vi "VI Server_GetComboBoxValuesArray.vi"(7 "Label":string, 8 "error in":errorcluster, 11 "VI Server Cluster":T1) -> (0 "error out":errorcluster, 1 "Control Reference":refnum<vi>, 3 "VI Server Custer.DUP":T1={"Labels"=["Label", "Size", "Font", "Heght", "Width", "Ledding Denominator", "Ledding Nominator", "Label Number", "Microstep Resolution", "X", "Y", "Z", "Italic?", "Underlined?"], "Refs"=[], "VI Ref"=refnum}, 4 "Strings[]":string[](array[string]), 6 "Values[]":string[](array[string]))   [LabVIEW 2020, in "VI Server Toolkit LV2013.lvlib"]
doc: "Returns array of item names and array of the corresponding values."
uses:
  VI Server Toolkit LV2013.lvlib
  VI Server_TypeDefs/VI Server_RefsCluster.ctl
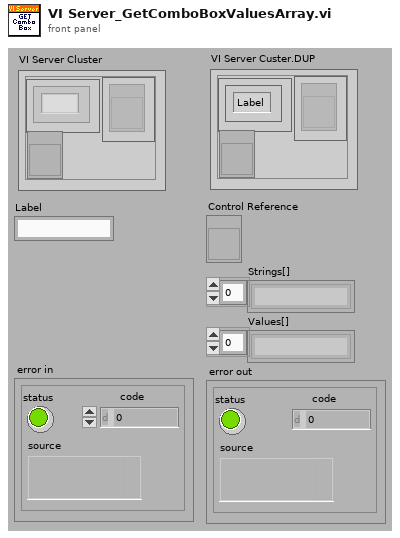
[diagram p1: front panel]
types:
  T1 = typedef "VI Server_RefsCluster.ctl" = cluster{"Labels":string[], "Refs":refnum<vi>[], "VI Ref":refnum<vi>}
  T2 = typedef "LVComboBoxStrsAndValuesArrayTypeDef.ctl" = cluster{"String":string, "Value":string}[]
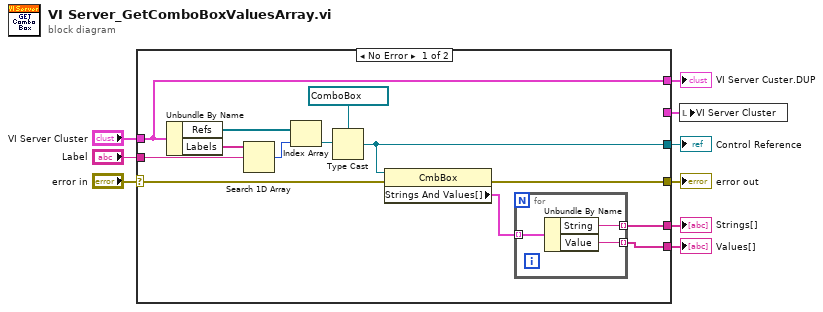
[diagram p0: block diagram]
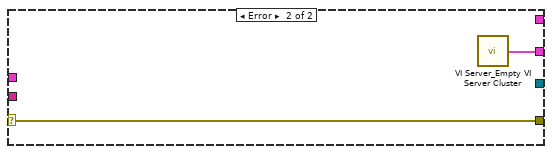
[diagram p2: hidden frame]
diagram:
  n1 = case shown="No Error" "error in" {
    selector: "error in" -> [w16 w27]
    tunnel: "Label" -> [w21 _]
    tunnel: "VI Server Cluster" -> [w10 _]
    tunnel: [w17 _] -> w5
    tunnel: [w15 w27] -> w9
    tunnel: [w12 _] -> w4
    tunnel: [w11 _] -> w3
    tunnel: [w10 _] -> w2
    tunnel: [_ w26] -> w1
    frame No Error {
      n2 = Unbundle By Name(w10) -> ("Refs"=w18:refnum<vi>[], "Labels"=w22:string[])
      n3 = Search 1D Array(1D array=w22, element=w21) -> (index of element=w20:i32)  [unwired: 1 out]
      n4 = Index Array(array=w18, index=w20) -> (element=w19:refnum<vi>)
      n5 = Type Cast(type=refnum<vi> refnum ("Default Value"), x=w19) -> (*(type *) &x=w17:refnum<vi>)
      n6 = property class="CmbBox"(reference=w17, error in=w16) -> (error out=w15:errorcluster, "Strings And Values[]"=w13:T2)  [unwired: 1 out]
      n7 = for {
        tunnel: w13 -> [w25] mode=indexing
        tunnel: [w24] -> w12 mode=indexing
        tunnel: [w23] -> w11 mode=indexing
        n8 = Unbundle By Name(w25) -> ("String"=w24:string, "Value"=w23:string)
      }
    }
    frame Error {
      n9 = call "VI Server_Empty VI Server Cluster.vi"() -> ("VI Server Cluster"=w26:T1)  [unwired: 7 in]
    }
  }
  "error out" <- w9
  "VI Server Custer.DUP" <- w2
  "Control Reference" <- w5
  "Strings[]" <- w4
  "Values[]" <- w3
  n10 = local write "VI Server Cluster"(w1) -> ()
